vi "number_with_decimal_points.vi"(6 "Precision":i16=6, 7 "Double":dbl=-8123456789.123456 format="%#.6f") -> (3 "String":string)   [LabVIEW 2025]
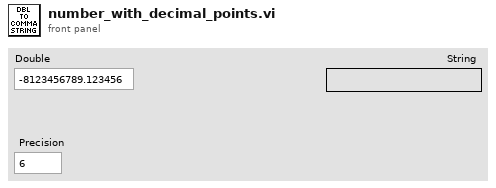
[diagram p1: front panel]
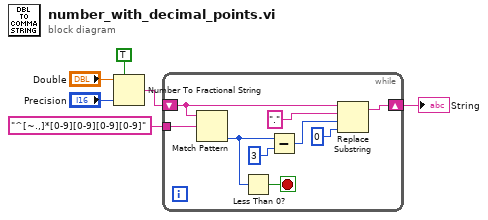
[diagram p0: block diagram]
diagram:
  n1 = Number To Fractional String(use system decimal point (T)=TRUE, number="Double", precision (6)="Precision") -> (F-format string=w2:string)  [unwired: 1 in]
  n2 = while {
    shift-right: [w7] -> w4
    shift-left: w2 -> [w9]
    tunnel: "^[~.,]*[0-9][0-9][0-9][0-9]" ("regular expression") -> [w12]
    stop <- w15 stop-if-true
    n3 = Match Pattern(string=w9, regular expression=w12) -> (offset past match=w8:i32)  [unwired: 1 in, 3 out]
    n4 = Less Than 0?(x=w8) -> (x < 0?=w15:bool)
    n5 = Subtract(x=w8, y=3) -> (x-y=w11:i32)
    n6 = Replace Substring(2:0 ("length (len. of substring)"), 3:w11, 4:"." ("substring (\"\")"), 5:w9) -> (1:w7:string)  [unwired: 1 out]
  }
  "String" <- w4
